vi "UHR-Fleezers Control (host) - 12.0_test_fpga_connection.vi"() -> ()   [LabVIEW 2014] (continued)
        n1069 = Multiply(x=w1416, y=w1429) -> (x*y=w1424:dbl)
        n1070 = Multiply(x=w1428, y=w1415) -> (x*y=w1422:dbl)
        n1071 = Multiply(x=w1427, y=w1414) -> (x*y=w1423:dbl)
        n1072 = Multiply(x=w1430, y=w1413) -> (x*y=w1433:dbl)
        n1073 = Multiply(x=w1431, y=w1412) -> (x*y=w1434:dbl)
        n1074 = Multiply(x=w1432, y=w1411) -> (x*y=w1435:dbl)
        n1075 = call "set RF board amplitude - interlace.vi"("Board 2 Amplitude Limits"=w1397, "Board 1 Amplitude Limits"=w1398, "error in"=w1425, "FPGA VI Reference In"=w1426, "Board 2 Amplitude 3 (%)"=w1435, "Board 1 Amplitude 3 (%)"=w1423, "Board 2 Amplitude 2 (%)"=w1434, "Board 2 Amplitude 1 (%)"=w1433, "Board 1 Amplitude 2 (%)"=w1422, "Board 1 Amplitude 1 (%)"=w1424) -> ("error out"=w1406:errorcluster, "FPGA VI Reference Out"=w1407:T22)
        n1076 = xnode "Read/Write Control"("FPGA VI Reference In"=w1407, "error in"=w1406, "FB On/Off Set 1"=w1402, "FB On/Off Set 2"=w1399) -> ("error out"=w1405:errorcluster)  [unwired: 1 out]
      }
      event "Load parameters": Value Change {
        n1077 = event-data() -> ()  [unwired: 7 out]
        n1078 = property on="Saved AOD Raster Scan Parameter Sets" class="Arr (strict)"() -> ("Index Values"=w1446:u32[])  [unwired: 2 in, 2 out]
        n1079 = Index Array(array=w1446, index=0) -> (element=w1443:u32)
        n1080 = local write "Load parameters"(FALSE ("Load parameters")) -> ()
        n1081 = Index Array(array="Saved AOD Raster Scan Parameter Sets", index=w1443) -> (element=w1442:T31)
        n1082 = Unbundle By Name(w1442) -> ("Scan Range AOD (nm) 2"=w1441:dbl, "Step Size AOD (nm) 2"=w1440:dbl, "Scan Speed AOD (nm/s) 2"=w1439:dbl, "Number of scans (AOD) 2"=w1438:u16)
        n1083 = flat-sequence {
          tunnel: w1441 -> [w1449]
          tunnel: w1440 -> [w1448]
          tunnel: w1439 -> [w1447]
          tunnel: w1438 -> [w1450]
          frame #0 {
            n1084 = local write "Scan Speed (nm/s)"(w1447) -> ()
            n1085 = local write "Scan Range (nm)"(w1449) -> ()
            n1086 = local write "Step Size (nm)"(w1448) -> ()
          }
          frame #1 {
            n1087 = property on="Number of F/B Scans (AOD)" class="DigNum (strict)"("Val(Sgnl)"=w1450) -> ()  [unwired: 2 in, 2 out]
          }
        }
      }
      event "Trap 1 (ON/OFF)", "Trap 2 (ON/OFF)": Value Change {
        n1088 = event-data() -> ()  [unwired: 7 out]
        n1089 = property on="Trap 2 ON" class="Bool (strict)"("Val(Sgnl)"="Trap 2 (ON/OFF)") -> ()  [unwired: 2 in, 2 out]
        n1090 = property on="Trap 1 ON" class="Bool (strict)"("Val(Sgnl)"="Trap 1 (ON/OFF)") -> ()  [unwired: 2 in, 2 out]
      }
      event "DIO count 1 (ticks)", "DIO count 2 (ticks)", "DIO count 3 (ticks)", "Interlace", "Number Interlace Sets", "Not-Interlacing Set": Value Change {
        n1091 = event-data() -> ()  [unwired: 7 out]
        n1092 = local read "DIO count 3 (ticks)"() -> (w1463:u32)
        n1093 = local read "DIO count 1 (ticks)"() -> (w1465:u32)
        n1094 = local read "DIO count 2 (ticks)"() -> (w1464:u32)
        n1095 = To Unsigned Byte Integer(number="Not-Interlacing Set") -> (unsigned 8bit integer=w1454:u8)
        n1096 = Add(x=w1454, y=u8 1) -> (x+y=w1458:u8)
        n1097 = xnode "Read/Write Control"("FPGA VI Reference In"=w1469, "error in"=w1467, "DIO count 1 (ticks)"=w1465, "DIO count 2 (ticks)"=w1464, "DIO count 3 (ticks)"=w1463, "Interlace ON/OFF"="Interlace", "Number Interlace Cycles"="Number Interlace Sets", "Interlace Off Parameters"=w1458) -> ("error out"=w1468:errorcluster)  [unwired: 1 out]
        n1098 = Build Array(w1465, w1464, w1463) -> (w1456:u32[])
        n1099 = Split 1D Array(array=w1456, index="Number Interlace Sets") -> (first subarray=w1466:u32[])  [unwired: 1 out]
        n1100 = Index Array(array=w1456, index=w1454) -> (element=w1455:u32)
        n1101 = Add Array Elements(numeric array=w1466) -> (sum=w1460:u32)
        n1102 = Select(t=w1460, s="Interlace", f=w1455) -> (s? t:f=→"Total Counts (ticks)":u32)
      }
      event "Reset Feedback": Value Change {
        n1103 = event-data() -> ()  [unwired: 7 out]
        n1104 = Unbundle By Name("Reset Feedback") -> ("Set 1"=w1473:bool, "Set 2"=w1472:bool)
        n1105 = xnode "Read/Write Control"("FPGA VI Reference In"=w1475, "error in"=w1470, "FB Reset Set 1"=w1473, "FB Reset Set 2"=w1472) -> ("error out"=w1471:errorcluster)  [unwired: 1 out]
      }
      event "PID Gains": Value Change {
        n1106 = event-data() -> ()  [unwired: 7 out]
        n1107 = Unbundle By Name("PID Gains") -> ("Set 1"=w1479:T15, "Set 2"=w1478:T15)
        n1108 = xnode "Read/Write Control"("FPGA VI Reference In"=w1480, "error in"=w1476, "FB Gains Set 1"=w1479, "FB Gains Set 2"=w1478) -> ("error out"=w1477:errorcluster)  [unwired: 1 out]
      }
      event "AI2 to Setpoint", "Setpoints (V)": Value Change {
        n1109 = event-data() -> ()  [unwired: 7 out]
        n1110 = xnode "Read/Write Control"("FPGA VI Reference In"=w1486, "error in"=w1482) -> ("FPGA VI Reference Out"=w1485:T22, "error out"=w1484:errorcluster, "AI2 Y Sum Set 1"=w1493:i16, "AI2 Y Sum Set 2"=w1492:i16)
        n1111 = Cluster To Array(cluster="AI2 to Setpoint") -> (array=w1496:bool[])
        n1112 = local read "AI2 (V)"() -> (w1494:cluster{"Set 1":dbl, "Set 2":dbl})
        n1113 = Or Array Elements(Boolean array=w1496) -> (logical OR=w1497:bool)
        n1114 = Bundle By Name(cluster=w1494, "Set 1"=w1493, "Set 2"=w1492) -> (w1491:cluster{"Set 1":dbl, "Set 2":dbl})
        n1115 = Divide(x=w1491, y=3276.7) -> (x/y=w1490:cluster{"Set 1":dbl, "Set 2":dbl})
        "AI2 (V)" <- w1490
        n1116 = case shown="True" w1497 {
          tunnel: [w1500 w1517] -> w1489
          tunnel: "AI2 to Setpoint" -> [_ w1513]
          tunnel: "Setpoints (V)" -> [w1501 w1516]
          tunnel: w1490 -> [_ w1510]
          frame False {
            n1117 = Multiply(x=3276.7, y=w1501) -> (x*y=w1502:cluster{"Set 1":dbl, "Set 2":dbl})
            n1118 = To Word Integer(number=w1502) -> (16bit integer=w1500:cluster{"Set 1":i16, "Set 2":i16})
          }
          frame True {
            n1119 = Unbundle By Name(w1510) -> ("Set 1"=w1509:dbl, "Set 2"=w1508:dbl)
            n1120 = Unbundle By Name(w1516) -> ("Set 1"=w1515:dbl, "Set 2"=w1514:dbl)
            n1121 = Unbundle By Name(w1513) -> ("Set 1"=w1512:bool, "Set 2"=w1511:bool)
            n1122 = Select(t=w1509, s=w1512, f=w1515) -> (s? t:f=w1507:dbl)
            n1123 = Select(t=w1508, s=w1511, f=w1514) -> (s? t:f=w1506:dbl)
            n1124 = Bundle By Name(cluster=w1516, "Set 1"=w1507, "Set 2"=w1506) -> (w1504:cluster{"Set 1":dbl, "Set 2":dbl})
            n1125 = local write "Setpoints (V)"(w1504) -> ()
            n1126 = Multiply(x=3276.7, y=w1504) -> (x*y=w1505:cluster{"Set 1":dbl, "Set 2":dbl})
            n1127 = To Word Integer(number=w1505) -> (16bit integer=w1517:cluster{"Set 1":i16, "Set 2":i16})
          }
        }
        n1128 = Unbundle By Name(w1489) -> ("Set 1"=w1488:i16, "Set 2"=w1487:i16)
        n1129 = xnode "Read/Write Control"("FPGA VI Reference In"=w1485, "error in"=w1484, "FB Setpoint Set 1"=w1488, "FB Setpoint Set 2"=w1487) -> ("error out"=w1483:errorcluster)  [unwired: 1 out]
      }
      event "Invert laser interlacing": Value Change {
        n1130 = event-data() -> ()  [unwired: 7 out]
        n1131 = xnode "Read/Write Control"("FPGA VI Reference In"=w1522, "error in"=w1520, "Invert GI"="Invert laser interlacing", "Invert GI 2"="Invert laser interlacing", "Invert RI"="Invert laser interlacing", "Invert RI 2"="Invert laser interlacing") -> ("error out"=w1521:errorcluster)  [unwired: 1 out]
      }
      event "Green FB Setpoint (mV)", "Green FB Gains", "Green FB On/Off", "Green intensity % (FB OFF)", "Green int current ON count adj", "Red intensity % (FB OFF)", "Red FB Gains", "Red FB On/Off", "Red FB Setpoint (mV)": Value Change {
        n1132 = event-data() -> ()  [unwired: 7 out]
        n1133 = local read "Green FB Setpoint (mV)"() -> (w1538:dbl)
        n1134 = local read "Green intensity % (FB OFF)"() -> (w1541:dbl)
        n1135 = local read "Red intensity % (FB OFF)"() -> (w1531:dbl)
        n1136 = local read "Red FB Setpoint (mV)"() -> (w1527:dbl)
        n1137 = Multiply(x=w1527, y=3.2767) -> (x*y=w1525:dbl)
        n1138 = Multiply(x=w1538, y=3.2767) -> (x*y=w1537:dbl)
        n1139 = Multiply(x=w1541, y=655.35) -> (x*y=w1542:dbl)
        n1140 = Multiply(x=w1531, y=655.35) -> (x*y=w1529:dbl)
        n1141 = To Unsigned Word Integer(number=w1542) -> (unsigned 16bit integer=w1540:u16)
        n1142 = To Unsigned Word Integer(number=w1529) -> (unsigned 16bit integer=w1528:u16)
        n1143 = local read "Green int current ON count adj"() -> (w1545:u16)
        n1144 = local read "Green FB Gains"() -> (w1544:T15)
        n1145 = local read "Laser interlacing mode (all lasers)"() -> (w1534:enum32{"Laser ON", "Laser OFF", "Interlace"})
        n1146 = local read "Green ON/Interlacing"() -> (w1535:bool)
        n1147 = local read "Red FB On/Off"() -> (w1524:bool)
        n1148 = local read "Green FB On/Off"() -> (w1546:bool)
        n1149 = local read "Red FB Gains"() -> (w1523:T15)
        n1150 = Equal?(x=w1534, y=enum32{"Laser ON", "Laser OFF", "Interlace"}."Interlace") -> (x = y?=w1532:bool)
        n1151 = Compound Arithmetic op=AND(w1532, w1546, w1535) -> (w1536:bool)
        n1152 = xnode "Read/Write Control"("FPGA VI Reference In"=w1549, "error in"=w1548, "Green FB Setpoint"=w1537, "Green FB On/Off"=w1536, "Current Out"=w1540, "Green int current ON count adj"=w1545, "Green FB Gains"=w1544, "RI Current Out"=w1528, "Red FB Setpoint"=w1525, "Red FB On/Off"=w1524, "Red FB Gains"=w1523) -> ("error out"=w1547:errorcluster)  [unwired: 1 out]
      }
      event "Laser interlacing mode (all lasers)", "Green ON/Interlacing", "Red Laser ON/Interlacing": Value Change {
        n1153 = event-data() -> ()  [unwired: 7 out]
        n1154 = local write "Green Laser ON/OFF"("Green ON/Interlacing") -> ()
        n1155 = case shown="True" "Green ON/Interlacing" {
          tunnel: "Laser interlacing mode (all lasers)" -> [_ w1573]
          tunnel: [enum32{"Laser ON", "Laser OFF", "Interlace"}."Laser OFF" ("Green laser mode") w1573] -> w1556
          tunnel: [FALSE w1569] -> w1555
          frame False {
          }
          frame True {
            n1156 = local read "Green FB On/Off"() -> (w1570:bool)
            n1157 = Equal?(x=w1573, y=enum32{"Laser ON", "Laser OFF", "Interlace"}."Interlace") -> (x = y?=w1571:bool)
            n1158 = And(x=w1571, y=w1570) -> (x .and. y?=w1569:bool)
          }
        }
        n1159 = case shown="True" "Red Laser ON/Interlacing" {
          tunnel: "Laser interlacing mode (all lasers)" -> [_ w1565]
          tunnel: [FALSE w1562] -> w1550
          tunnel: [enum32{"Laser ON", "Laser OFF", "Interlace"}."Laser OFF" ("Green laser mode") w1565] -> w1551
          frame False {
          }
          frame True {
            n1160 = local read "Red FB On/Off"() -> (w1563:bool)
            n1161 = Equal?(x=w1565, y=enum32{"Laser ON", "Laser OFF", "Interlace"}."Interlace") -> (x = y?=w1564:bool)
            n1162 = And(x=w1564, y=w1563) -> (x .and. y?=w1562:bool)
          }
        }
        n1163 = xnode "Read/Write Control"("FPGA VI Reference In"=w1559, "error in"=w1557, "Operating Mode"=w1556, "Operating Mode 2"=w1556, "Green FB On/Off"=w1555, "Red operating mode"=w1551, "RI operating mode 2"=w1551, "Red FB On/Off"=w1550) -> ("error out"=w1558:errorcluster)  [unwired: 1 out]
      }
      event "Green Laser ON/OFF": Value Change {
        n1164 = event-data() -> ()  [unwired: 7 out]
        n1165 = property on="Green ON/Interlacing" class="Bool (strict)"("Val(Sgnl)"="Green Laser ON/OFF") -> ()  [unwired: 2 in, 2 out]
      }
      event "Test ttrig": Value Change {
        n1166 = event-data() -> ()  [unwired: 7 out]
        n1167 = xnode "Read/Write Control"("FPGA VI Reference In"=w1578, "error in"=w1577, "TTrig?"=TRUE) -> ("error out"=w1576:errorcluster)  [unwired: 1 out]
      }
      event "Neg. TTrig FPGA": Value Change {
        n1168 = event-data() -> ()  [unwired: 7 out]
        n1169 = xnode "Read/Write Control"("FPGA VI Reference In"=w1582, "error in"=w1581, "TTrig Negate Pos"="Neg. TTrig FPGA") -> ()  [unwired: 2 out]
      }
      event "- phase (APD 1 Gate)", "+ phase (APD 1 Gate)": Value Change {
        n1170 = event-data() -> ()  [unwired: 7 out]
        n1171 = local read "Phase Adj. (APD 1 Gate)"() -> (w1583:i16)
        n1172 = Negate(x=w1583) -> (-x=w1591:i16)
        n1173 = Select(t=w1591, s="- phase (APD 1 Gate)", f=w1583) -> (s? t:f=w1590:i16)
        n1174 = Or(x="- phase (APD 1 Gate)", y="+ phase (APD 1 Gate)") -> (x .or. y?=w1586:bool)
        n1175 = xnode "Read/Write Control"("FPGA VI Reference In"=w1593, "error in"=w1592, "Phase count adjustment (APD 1 Gate)"=w1590) -> ("FPGA VI Reference Out"=w1588:T22, "error out"=w1589:errorcluster)
        n1176 = xnode "Read/Write Control"("FPGA VI Reference In"=w1588, "error in"=w1589, "+ phase (APD 1 Gate)"=w1586) -> ("error out"=w1587:errorcluster)  [unwired: 1 out]
      }
      event "+ phase (APD 2 Gate)", "- phase (APD 2 Gate)": Value Change {
        n1177 = event-data() -> ()  [unwired: 7 out]
        n1178 = local read "Phase Adj. (APD 2 Gate)"() -> (w1594:i16)
        n1179 = Negate(x=w1594) -> (-x=w1602:i16)
        n1180 = Select(t=w1602, s="- phase (APD 2 Gate)", f=w1594) -> (s? t:f=w1601:i16)
        n1181 = Or(x="- phase (APD 2 Gate)", y="+ phase (APD 2 Gate)") -> (x .or. y?=w1597:bool)
        n1182 = xnode "Read/Write Control"("FPGA VI Reference In"=w1604, "error in"=w1603, "Phase count adjustment (APD 2 Gate)"=w1601) -> ("FPGA VI Reference Out"=w1599:T22, "error out"=w1600:errorcluster)
        n1183 = xnode "Read/Write Control"("FPGA VI Reference In"=w1599, "error in"=w1600, "+ phase (APD 2 Gate)"=w1597) -> ("error out"=w1598:errorcluster)  [unwired: 1 out]
      }
      event "Phase Adj. (APD Acq)", "+ phase (APD Acq)", "- phase (APD Acq)": Value Change {
        n1184 = event-data() -> ()  [unwired: 7 out]
        n1185 = local read "Phase Adj. (APD Acq)"() -> (w1607:i16)
        n1186 = Negate(x=w1607) -> (-x=w1613:i16)
        n1187 = Select(t=w1613, s="+ phase (APD Acq)", f=w1607) -> (s? t:f=w1612:i16)
        n1188 = Or(x="+ phase (APD Acq)", y="- phase (APD Acq)") -> (x .or. y?=w1608:bool)
        n1189 = xnode "Read/Write Control"("FPGA VI Reference In"=w1615, "error in"=w1614, "Phase Count Adjustment (APD Acq)"=w1612) -> ("FPGA VI Reference Out"=w1610:T22, "error out"=w1611:errorcluster)
        n1190 = xnode "Read/Write Control"("FPGA VI Reference In"=w1610, "error in"=w1611, "+ phase (APD Acq)"=w1608) -> ("error out"=w1609:errorcluster)  [unwired: 1 out]
      }
      event "Phase adj. (GI)", "+ phase (GI)", "- phase (GI)", "+phase (RI)", "- phase (RI)", "Phase adj. (RI)": Value Change {
        n1191 = event-data() -> ()  [unwired: 7 out]
        n1192 = Negate(x="Phase adj. (GI)") -> (-x=w1630:i16)
        n1193 = Select(t=w1630, s="+ phase (GI)", f="Phase adj. (GI)") -> (s? t:f=w1629:i16)
        n1194 = Or(x="+ phase (GI)", y="- phase (GI)") -> (x .or. y?=w1625:bool)
        n1195 = Negate(x="Phase adj. (RI)") -> (-x=w1620:i16)
        n1196 = Select(t=w1620, s="+phase (RI)", f="Phase adj. (RI)") -> (s? t:f=w1617:i16)
        n1197 = Or(x="+phase (RI)", y="- phase (RI)") -> (x .or. y?=w1616:bool)
        n1198 = xnode "Read/Write Control"("FPGA VI Reference In"=w1632, "error in"=w1631, "Phase count adjustment (GI)"=w1629, "Phase count adjustment (RI)"=w1617) -> ("FPGA VI Reference Out"=w1627:T22, "error out"=w1628:errorcluster)
        n1199 = xnode "Read/Write Control"("FPGA VI Reference In"=w1627, "error in"=w1628, "+ phase (GI)"=w1625, "+ phase (RI)"=w1616) -> ("error out"=w1626:errorcluster)  [unwired: 1 out]
      }
      event "+ phase (GI) 2", "- phase (GI) 2": Value Change {
        n1200 = event-data() -> ()  [unwired: 7 out]
        n1201 = Negate(x="Phase adj. (GI) 2") -> (-x=w1641:i16)
        n1202 = Select(t=w1641, s="+ phase (GI) 2", f="Phase adj. (GI) 2") -> (s? t:f=w1640:i16)
        n1203 = Or(x="+ phase (GI) 2", y="- phase (GI) 2") -> (x .or. y?=w1636:bool)
        n1204 = xnode "Read/Write Control"("FPGA VI Reference In"=w1643, "error in"=w1642, "Phase count adjustment (GI) 2"=w1640) -> ("FPGA VI Reference Out"=w1638:T22, "error out"=w1639:errorcluster)
        n1205 = xnode "Read/Write Control"("FPGA VI Reference In"=w1638, "error in"=w1639, "+ phase (GI) 2"=w1636) -> ("error out"=w1637:errorcluster)  [unwired: 1 out]
      }
      event "Phase adj. (Green FB)", "- phase (Green FB)", "+ phase (Green FB)": Value Change {
        n1206 = event-data() -> ()  [unwired: 7 out]
        n1207 = Negate(x="Phase adj. (Green FB)") -> (-x=w1652:i16)
        n1208 = Select(t=w1652, s="+ phase (Green FB)", f="Phase adj. (Green FB)") -> (s? t:f=w1651:i16)
        n1209 = Or(x="+ phase (Green FB)", y="- phase (Green FB)") -> (x .or. y?=w1647:bool)
        n1210 = xnode "Read/Write Control"("FPGA VI Reference In"=w1654, "error in"=w1653, "Phase count adjustment (Green FB)"=w1651) -> ("FPGA VI Reference Out"=w1649:T22, "error out"=w1650:errorcluster)
        n1211 = xnode "Read/Write Control"("FPGA VI Reference In"=w1649, "error in"=w1650, "+ phase (Green FB)"=w1647) -> ("error out"=w1648:errorcluster)  [unwired: 1 out]
      }
      event "Invert APD Gate", "APD Gate ON Count", "APD Gate OFF Count", "APD Gate", "APD Integration Time (s)", "APD 1 AO Mult.", "APD 2 AO Mult.", "Duty frequency (ON 1/N cycles)": Value Change {
        n1212 = event-data() -> ()  [unwired: 7 out]
        n1213 = Add(x="Interlace ON count", y="Interlace OFF count") -> (x+y=w1658:u16)
        n1214 = Add(x="APD Gate ON Count", y="APD Gate OFF Count") -> (x+y=w1671:u16)
        n1215 = Multiply(x="Duty frequency (ON 1/N cycles)", y=w1658) -> (x*y=w1657:u16)
        "Green FB Count" <- w1657
        n1216 = Subtract(x=w1657, y="Interlace ON count") -> (x-y=w1655:u16)
        n1217 = Multiply(x=w1671, y="Duty frequency (ON 1/N cycles)") -> (x*y=w1670:u16)
        n1218 = Subtract(x=w1670, y="APD Gate ON Count") -> (x-y=w1669:u16)
        n1219 = local read "DMA Update Period (s)"() -> (w1672:dbl)
        n1220 = Multiply(x="APD Integration Time (s)", y=40000000.0) -> (x*y=w1677:dbl)
        n1221 = Reciprocal(x="APD Integration Time (s)") -> (1/x=→"APD Acq Rate (Hz)":dbl)
        n1222 = To Unsigned Long Integer(number=w1677) -> (unsigned 32bit integer=w1661:u32)
        "APD Int. Count" <- w1661
        n1223 = xnode "Read/Write Control"("FPGA VI Reference In"=w1681, "error in"=w1680, "Invert APD Gate"="Invert APD Gate", "APD Gate ON Count"="APD Gate ON Count", "APD Gate OFF Count"=w1669, "APD Acq Rate Count"=w1661, "APD Gate Operating Mode"="APD Gate", "APD 1 AO scale factor"="APD 1 AO Mult.", "APD 2 AO scale factor"="APD 2 AO Mult.", "Green interlace ON count"="Interlace ON count", "Green interlace OFF count"=w1655, "Green interlace ON count 2"="Interlace ON count", "Green interlace OFF count 2"=w1655, "Green FB Count"=w1657, "RI ON count"="Interlace ON count", "RI OFF count"=w1655) -> ("error out"=w1679:errorcluster)  [unwired: 1 out]
        n1224 = Divide(x=w1672, y="APD Integration Time (s)") -> (x/y=w1675:dbl)
        n1225 = Multiply(x=2.0, y=w1675) -> (x*y=w1674:dbl)
        n1226 = local write "APD Samples/FIFO Acq."(w1675) -> ()
        n1227 = local write "APD Elements/DMA read"(w1674) -> ()
      }
      event "Number of F/B Scans (AOD)", "Scan Speed (nm/s)", "Scan BD", "Initial D (MHz)", "Step Size (nm)", "Scan Range (nm)", "Wiggle amp 1 (units?)": Value Change {
        w1743 = 123.0  # AOM cal (nm/MHz)
        n1228 = event-data() -> ()  [unwired: 7 out]
        n1229 = local read "BD 1 Frequency 1 (MHz)"() -> (w1726:dbl)
        n1230 = local read "AOM X Cal (nm/MHz)"() -> (w1718:dbl)
        n1231 = local read "BD 2 Frequency 1 (MHz)"() -> (w1732:dbl)
        n1232 = local read "X RF Frequency Limits (MHz)"() -> (w1730:T17)
        n1233 = local read "Y RF Frequency Limits (MHz)"() -> (w1727:T17)
        n1234 = Negate(x="Scan Range (nm)") -> (-x=w1696:dbl)
        n1235 = Divide(x=w1696, y=w1718) -> (x/y=w1700:dbl)
        n1236 = Select(t=w1730, s="Scan BD", f=w1727) -> (s? t:f=w1729:T17)
        n1237 = Select(t=w1726, s="Scan BD", f=w1732) -> (s? t:f=w1731:dbl)
        n1238 = Unbundle By Name(w1729) -> ("Maximum"=w1738:dbl, "Minimum"=w1737:dbl)
        n1239 = Add(x=w1700, y=w1731) -> (x+y=w1735:dbl)
        n1240 = Divide(x=w1696, y="Step Size (nm)") -> (x/y=w1715:dbl)
        n1241 = Divide(x="Step Size (nm)", y=w1718) -> (x/y=w1724:dbl)
        n1242 = Absolute Value(x=w1715) -> (abs(x)=w1699:dbl)
        n1243 = Sign(1:w1696) -> (0:w1697:dbl)
        n1244 = In Range and Coerce(upper limit=w1738, x=w1735, lower limit=w1737) -> (coerced(x)=w1734:dbl, In Range?=w1736:bool)
        n1245 = To Unsigned Quad Integer(1:w1699) -> (0:w1714:u64)
        "Scan steps (AOD)" <- w1714
        n1246 = call "IR AOM freq to word.vi"("Frequency In (MHz)"=w1724) -> ("Frequency Word Out (double)"=w1721:dbl)
        n1247 = Multiply(x=w1697, y=w1721) -> (x*y=w1698:dbl)
        n1248 = Subtract(x=w1735, y=w1734) -> (x-y=w1733:dbl)
        n1249 = To Quad Integer(1:w1698) -> (0:w1720:i64)
        "Incr. int (AOD)" <- w1720
        n1250 = Subtract(x=w1700, y=w1733) -> (x-y=w1719:dbl)
        "Scan Range (MHz)" <- w1719
        n1251 = Select(t=w1700, s=w1736, f=w1719) -> (s? t:f=w1739:dbl)
        n1252 = Multiply(x=w1719, y=w1718) -> (x*y=w1717:dbl)
        n1253 = Decrement(x=w1714) -> (x-1=w1767:u64)
        n1254 = Negate(x=w1717) -> (-x=w1713:dbl)
        n1255 = local write "Scan Range (nm)"(w1713) -> ()
        n1256 = Divide(x=w1739, y=w1767) -> (x/y=w1723:dbl)
        "Scan Increment (MHz)" <- w1723
        n1257 = call "IR AOM freq to word.vi"("Frequency In (MHz)"=w1723) -> ("Frequency Word Out (double)"=w1722:dbl)
        n1258 = Divide(x="Step Size (nm)", y="Scan Speed (nm/s)") -> (x/y=w1710:dbl)
        n1259 = To Quad Integer(1:w1722) -> ()  [unwired: 1 out]
        n1260 = local read "Number Interlace Sets"() -> (w1694:u8)
        n1261 = local read "AI Count (ticks)"() -> (w1695:u32)
        n1262 = local read "Total Counts (ticks)"() -> (w1693:u32)
        n1263 = local read "# Samples/trap"() -> (w1725:u32)
        n1264 = Multiply(x=w1695, y=w1694) -> (x*y=w1692:u32)
        n1265 = Divide(x=w1693, y=w1692) -> (x/y=w1691:dbl)
        n1266 = Select(t=w1726, s="Scan BD", f=w1732) -> (s? t:f=w1764:dbl)
        "Initial freq. (MHz)" <- w1764
        n1267 = Add(x=w1739, y=w1764) -> (x+y=→"Final freq. (MHz)":dbl)
        n1268 = Divide(x=w1693, y=40000000.0) -> (x/y=w1709:dbl)
        n1269 = Divide(x=w1710, y=w1709) -> (x/y=w1708:dbl)
        n1270 = To Unsigned Quad Integer(1:w1708) -> (0:w1683:u64)
        n1271 = Quotient & Remainder(x=w1683, y=u64 2) -> (x-y*floor(x/y)=w1687:u64)  [unwired: 1 out]
        n1272 = Equal?(x=w1687, y=u64 0) -> (x = y?=w1685:bool)
        n1273 = Decrement(x=w1683) -> (x-1=w1684:u64)
        n1274 = Select(t=w1683, s=w1685, f=w1684) -> (s? t:f=w1682:u64)
        "Cycles/step (AOD)" <- w1682
        n1275 = xnode "Read/Write Control"("FPGA VI Reference In"=w1775, "error in"=w1774, "Scan steps"=w1714, "Number of scans"="Number of F/B Scans (AOD)", "Cycles per step"=w1682, "Scan freq.  increment"=w1720, "Scan BD"="Scan BD") -> ("error out"=w1773:errorcluster)  [unwired: 1 out]
        n1276 = Multiply(x=w1714, y=w1682) -> (x*y=w1768:u64)
        n1277 = Multiply(x=w1768, y=u64 2) -> (x*y=w1690:u64)
        n1278 = Multiply(x=w1691, y=w1690) -> (x*y=w1689:dbl)
        "Data points/scan (f/b)" <- w1689
        n1279 = Multiply(x=w1689, y="Number of F/B Scans (AOD)") -> (x*y=w1771:dbl)
        "Data points/scans" <- w1771
        n1280 = Divide(x=w1771, y=w1725) -> (x/y=→"N sets should be saved":dbl)
        n1281 = Multiply(x=w1768, y=w1709) -> (x*y=w1707:dbl)
        "Time/Scan (s) (AOD)" <- w1707
        n1282 = Select(t=w1739, s="Scan BD", f=0.0) -> (s? t:f=w1765:dbl)
        n1283 = Select(t=0.0, s="Scan BD", f=w1739) -> (s? t:f=w1761:dbl)
        n1284 = local read "BD 2 Frequency 2 (MHz)"() -> (w1757:dbl)
        n1285 = local read "BD 1 Frequency 2 (MHz)"() -> (w1760:dbl)
        n1286 = Add(x=w1761, y=w1732) -> (x+y=w1758:dbl)
        n1287 = Add(x=w1726, y=w1765) -> (x+y=w1759:dbl)
        n1288 = Multiply(x=w1707, y=2.0) -> (x*y=w1706:dbl)
        n1289 = Multiply(x=w1706, y="Number of F/B Scans (AOD)") -> (x*y=w1703:dbl)
        n1290 = Divide(x=w1703, y=60.0) -> (x/y=→"Time to Finish All (min)":dbl)
        n1291 = Add(x="Trap 2 Bead Size (nm)", y="Trap 1 Bead Size (nm)") -> (x+y=w1747:dbl)
        n1292 = Divide(x=w1747, y=2.0) -> (x/y=w1741:dbl)
        n1293 = Subtract(x=w1758, y=w1757) -> (x-y=w1755:dbl)
        n1294 = Subtract(x=w1759, y=w1760) -> (x-y=w1756:dbl)
        n1295 = local read "Initial D (MHz)"() -> (w1744:dbl)
        n1296 = Square(x=w1755) -> (x^2=w1754:dbl)
        n1297 = Square(x=w1756) -> (x^2=w1753:dbl)
        n1298 = Add(x=w1753, y=w1754) -> (x+y=w1752:dbl)
        n1299 = Square Root(x=w1752) -> (sqrt(x)=w1751:dbl)
        "Final D (MHz)" <- w1751
        n1300 = Multiply(x=w1743, y=w1751) -> (x*y=w1750:dbl)
        n1301 = Multiply(x=w1744, y=w1743) -> (x*y=w1742:dbl)
        n1302 = Subtract(x=w1742, y=w1741) -> (x-y=→"Initial sep (nm)":dbl)
        n1303 = Subtract(x=w1750, y=w1741) -> (x-y=→"Final sep (nm)":dbl)
      }
      event "Freq or Amp switch first", "Swap F1 and F2", "Freq switch delay", "Amp switch delay": Value Change {
        n1304 = event-data() -> ()  [unwired: 7 out]
        n1305 = local read "Freq or Amp switch first"() -> (w1776:bool)
        n1306 = local read "Amp switch delay"() -> (w1777:u16)
        n1307 = local read "Freq switch delay"() -> (w1779:u16)
        n1308 = local read "Swap F1 and F2"() -> (w1778:bool)
        n1309 = xnode "Read/Write Control"("FPGA VI Reference In"=w1782, "error in"=w1781, "Freq switch delay"=w1779, "Swap F1 and F2"=w1778, "Amp switch delay"=w1777, "Freq or Amp switch first"=w1776) -> ("error out"=w1780:errorcluster)  [unwired: 1 out]
      }
      event "Scan steps (MCL)", "Number of scans (MCL)", "Scan Range (V)\n(of steps)", "2D or 1D Scan", "N APD Samp/step", "Fast Scan Dir", "Continuous MCL Scanning", "Scan lines (y)": Value Change {
        w1784 = 32767.0 ("y")
        n1310 = event-data() -> ()  [unwired: 7 out]
        n1311 = Select(t="Scan lines (y)", s="2D or 1D Scan", f="Number of scans (MCL)") -> (s? t:f=w1789:u64)
        n1312 = Decrement(x="Scan steps (MCL)") -> (x-1=w1805:u64)
        n1313 = Divide(x="Scan Range (V)\n(of steps)", y=w1805) -> (x/y=w1804:dbl)
        "Desired Scan Incr (V)" <- w1804
        n1314 = local read "APD Integration Time (s)"() -> (w1797:dbl)
        n1315 = Multiply(x=w1804, y=w1784) -> (x*y=w1813:dbl)
        n1316 = Divide(x=w1813, y=10.0) -> (x/y=w1803:dbl)
        "Desired incr (int)" <- w1803
        n1317 = local read "Update Count (MCL)"() -> (w1809:u32)
        n1318 = Round Toward -Infinity(1:w1803) -> (0:w1812:dbl)
        n1319 = To Word Integer(number=w1812) -> (16bit integer=w1787:i16)
        "Actual Incr. int (MCL)" <- w1787
        n1320 = Multiply(x=w1797, y=40000000.0) -> (x*y=w1810:dbl)
        n1321 = Divide(x=w1810, y=w1809) -> (x/y=w1808:dbl)
        n1322 = Multiply(x=i16 10, y=w1787) -> (x*y=w1785:i16)
        n1323 = Multiply(x="N APD Samp/step", y=w1808) -> (x*y=w1807:dbl)
        "Cycles/step (MCL)" <- w1807
        n1324 = Divide(x=w1785, y=w1784) -> (x/y=→"Actual MCL Inc (V)":dbl)
        n1325 = Multiply(x="N APD Samp/step", y="Scan steps (MCL)") -> (x*y=w1799:dbl)
        n1326 = local read "APD Samples/FIFO Acq."() -> (w1796:dbl)
        n1327 = Multiply(x=w1799, y=u64 2) -> (x*y=w1798:dbl)
        "Data points/scan (f+b)" <- w1798
        n1328 = Multiply(x=w1798, y=w1789) -> (x*y=w1816:dbl)
        "Data points/scans (MCL)" <- w1816
        n1329 = Multiply(x=w1797, y=w1798) -> (x*y=w1790:dbl)
        "Time/f+b scan (s) (MCL)" <- w1790
        n1330 = Divide(x=w1816, y=w1796) -> (x/y=→"N sets should be saved (MCL)":dbl)
        n1331 = Multiply(x=w1790, y=w1789) -> (x*y=→"Total Time (s)":dbl)
        n1332 = Not(x="Fast Scan Dir") -> (.not. x?=w1794:bool)
        n1333 = xnode "Read/Write Control"("FPGA VI Reference In"=w1820, "error in"=w1819, "Scan steps (MCL)"="Scan steps (MCL)", "Number of scans (MCL)"=w1789, "Cycles per step (MCL)"=w1807, "Scan freq.  increment (MCL)"=w1787, "1D or 2D Scan?"="2D or 1D Scan", "MCL Scan Axis"=w1794, "Cont. Scan (MCL)"="Continuous MCL Scanning") -> ("error out"=w1818:errorcluster)  [unwired: 1 out]
      }
      event "Read Cal": Value Change {
        w1822 = 1000.0 ("y")
        n1334 = event-data() -> ()  [unwired: 7 out]
        n1335 = local read "Save file name"() -> (w1847:path)
        n1336 = local write "Read Cal"(FALSE ("Read Cal")) -> ()
        n1337 = Strip Path(path=w1847) -> (stripped path=w1846:path)  [unwired: 1 out]
        n1338 = Path To String(path=w1846) -> (string=w1845:string)
        n1339 = Concatenate Strings(w1845, "\\current.cal" ("string")) -> (w1843:string)
        n1340 = String To Path(string=w1843) -> (path=w1842:path)
        n1341 = Open/Create/Replace File(file path (use dialog)=w1842, operation (0:open)=T30."open", access (0:read/write)=enum16{"read/write", "read-only", "write-only"}."read-only") -> (refnum out=w1850:refnum<file>, error out=w1836:errorcluster)  [unwired: 1 in, 3 out]
        n1342 = Deny Access(4:w1836, 7:w1850) -> (0:w1835:errorcluster, 3:w1841:refnum<file>)  [unwired: 1 out]
        n1343 = Read from Binary File(5:0.0, 8:w1835, 9:T29."big-endian, network order" ("byte order (0:big-endian, network order)"), 10:-1 ("count (1)"), 11:w1841) -> (0:w1834:errorcluster, 2:w1832:dbl[], 3:w1837:refnum<file>)  [unwired: 2 out]
        n1344 = Array To Cluster(array=w1832) -> (cluster=w1831:T32)
        n1345 = Unbundle(w1831) -> ("[0]"=w1830:dbl, "[1]"=w1829:dbl, "[2]"=w1828:dbl, "[3]"=w1827:dbl, "[4]"=w1826:dbl, "[5]"=w1825:dbl)
        n1346 = Close File(refnum=w1837, error in=w1834) -> (error out=→"Read cal error":errorcluster)  [unwired: 1 out]
        n1347 = Multiply(x=w1825, y=w1822) -> (x*y=w1823:dbl)
        n1348 = local write "T2 k_x (pN/nm)"(w1827) -> ()
        n1349 = local write "T1 k_x (pN/nm)"(w1828) -> ()
        n1350 = local write "T1 a_x (nm/V)"(w1830) -> ()
        n1351 = local write "T2 a_x (nm/V)"(w1829) -> ()
        n1352 = Multiply(x=w1826, y=w1822) -> (x*y=w1824:dbl)
        n1353 = local write "T1 offset_x (mV)"(w1824) -> ()
        n1354 = local write "T2 offset_x (mV)"(w1823) -> ()
      }
      event "Read FX file": Value Change {
        n1355 = event-data() -> ()  [unwired: 7 out]
        n1356 = local write "Read FX file"(FALSE ("Read residual")) -> ()
        n1357 = local read "Save file name"() -> (w1875:path)
        n1358 = Strip Path(path=w1875) -> (stripped path=w1874:path)  [unwired: 1 out]
        n1359 = Path To String(path=w1874) -> (string=w1873:string)
        n1360 = Concatenate Strings(w1873, "\\current.cal" ("string")) -> (w1871:string)
        n1361 = String To Path(string=w1871) -> (path=w1870:path)
        n1362 = Open/Create/Replace File(file path (use dialog)=w1870, operation (0:open)=T30."open", access (0:read/write)=enum16{"read/write", "read-only", "write-only"}."read-only") -> (refnum out=w1867:refnum<file>, error out=w1864:errorcluster)  [unwired: 3 in, 1 out]
        n1363 = Deny Access(4:w1864, 7:w1867) -> (0:w1863:errorcluster, 3:w1866:refnum<file>)  [unwired: 1 in]
        n1364 = Read from Binary File(5:0.0, 8:w1863, 9:T29."big-endian, network order" ("byte order (0:big-endian, network order)"), 10:-1 ("count"), 11:w1866) -> (0:w1859:errorcluster, 2:w1853:dbl[], 3:w1860:refnum<file>)  [unwired: 1 in, 1 out]
        n1365 = Index Array(array=w1853, index=6) -> (element=→"Bad fit error":dbl)
        n1366 = Index Array(array=w1853, index=7) -> (element=→"Fit offset":dbl)
        n1367 = Index Array(array=w1853, index=8) -> (element=→"Hyst. error":dbl)
        n1368 = Close File(refnum=w1860, error in=w1859) -> ()  [unwired: 2 out]
      }
      event "Abort MCL Scan": Value Change {
        n1369 = event-data() -> ()  [unwired: 7 out]
        n1370 = local write "MCL Scanning"(FALSE ("MCL Scanning")) -> ()
        n1371 = xnode "Read/Write Control"("FPGA VI Reference In"=w1880, "error in"=w1879, "Abort scan (MCL)"="Abort MCL Scan") -> ("error out"=w1878:errorcluster)  [unwired: 1 out]
      }
      event "Update Count (MCL)": Value Change {
        n1372 = event-data() -> ()  [unwired: 7 out]
        n1373 = xnode "Read/Write Control"("FPGA VI Reference In"=w1884, "error in"=w1883, "MCL count"="Update Count (MCL)") -> ("error out"=w1882:errorcluster)  [unwired: 1 out]
      }
      event "Phase adjust (MCL)", "+ phase (MCL)", "- phase (MCL)": Value Change {
        n1374 = event-data() -> ()  [unwired: 7 out]
        n1375 = Negate(x="Phase adjust (MCL)") -> (-x=w1893:i16)
        n1376 = Select(t=w1893, s="- phase (MCL)", f="Phase adjust (MCL)") -> (s? t:f=w1891:i16)
        n1377 = Or(x="- phase (MCL)", y="+ phase (MCL)") -> (x .or. y?=w1886:bool)
        n1378 = xnode "Read/Write Control"("FPGA VI Reference In"=w1895, "error in"=w1894, "Phase count adjustment (MCL)"=w1891) -> ("FPGA VI Reference Out"=w1887:T22, "error out"=w1888:errorcluster)
        n1379 = xnode "Read/Write Control"("FPGA VI Reference In"=w1887, "error in"=w1888, "+ phase (MCL)"=w1886) -> ("error out"=w1885:errorcluster)  [unwired: 1 out]
      }
      event "Abort AOD Scan": Value Change {
        n1380 = event-data() -> ()  [unwired: 7 out]
        n1381 = xnode "Read/Write Control"("FPGA VI Reference In"=w1899, "error in"=w1898, "Abort scan"="Abort AOD Scan") -> ("error out"=w1897:errorcluster)  [unwired: 1 out]
      }
      event "Continuous AOD Scanning": Value Change {
        n1382 = event-data() -> ()  [unwired: 7 out]
        n1383 = xnode "Read/Write Control"("FPGA VI Reference In"=w1903, "error in"=w1902, "Cont. Scan"="Continuous AOD Scanning") -> ("error out"=w1901:errorcluster)  [unwired: 1 out]
      }
      event "Index": Value Change {
        n1384 = event-data() -> ()  [unwired: 7 out]
        n1385 = call "Create new save file.vi"("Insert"="", "Ext"=".dat" ("string"), "Index In"="Index") -> ("Path Out"=→"Save file name":path, "Index Out"=w1904:dbl)
        "Save index" <- w1904
        n1386 = local write "Index"(w1904) -> ()
      }
      event "AO1", "AO2": Value Change {
        w1919 = 10.0 ("y")
        w1918 = 32767.0 ("y")
        n1387 = event-data() -> ()  [unwired: 7 out]
        n1388 = local read "AO2"() -> (w1917:dbl)
        n1389 = local read "AO1"() -> (w1914:dbl)
        n1390 = Multiply(x=w1914, y=w1918) -> (x*y=w1913:dbl)
        n1391 = Multiply(x=w1917, y=w1918) -> (x*y=w1916:dbl)
        n1392 = Divide(x=w1913, y=w1919) -> (x/y=w1912:dbl)
        n1393 = Divide(x=w1916, y=w1919) -> (x/y=w1915:dbl)
        n1394 = To Word Integer(number=w1912) -> (16bit integer=w1920:i16)
        n1395 = To Word Integer(number=w1915) -> (16bit integer=w1921:i16)
        n1396 = xnode "Read/Write Control"("FPGA VI Reference In"=w1911, "error in"=w1910, "AO1"=w1920, "AO2"=w1921) -> ("error out"=w1909:errorcluster)  [unwired: 1 out]
      }
      event "Inject Pump 1": Value Change {
        n1397 = event-data() -> ()  [unwired: 7 out]
        n1398 = local read "Use Harvard pumps\nfor beads (else Chemyx)"() -> (w1923:bool)
        n1399 = case shown="True" w1923 {
          tunnel: "Inject Pump 1" -> [w1927 w1965]
          tunnel: w1922 -> [_ w1966]
          frame False {
            n1400 = local read "Pump write delay (ms)"() -> (w1926:dbl)
            n1401 = local read "Chemyx Syringe Pump Serial Port"() -> (w1925:refnum<visa-resource-name>)
            n1402 = case shown="True" w1927 {
              tunnel: w1926 -> [w1933 w1947]
              tunnel: w1925 -> [w1930 w1946]
              frame False {
                n1403 = flat-sequence {
                  tunnel: w1930 -> [w1934]
                  tunnel: [w1934] -> w1931
                  tunnel: w1933 -> [_]
                  tunnel: [w1937] -> w1932
                  tunnel: w1931 -> [w1937]
                  tunnel: w1932 -> [w1938]
                  tunnel: [w1938] -> w1928
                  tunnel: [w1940] -> w1929
                  tunnel: w1928 -> [w1940]
                  tunnel: w1929 -> [w1942]
                  frame #0 {
                    n1404 = call "Write to pump.vi"("string"="enter pump1", "VISA resource name"=w1934) -> ()  [unwired: 1 out]
                  }
                  frame #1 {
                    n1405 = Wait (ms)(milliseconds to wait="Pump pause delay (ms)") -> ()  [unwired: 1 out]
                  }
                  frame #2 {
                    n1406 = call "Write to pump.vi"("string"="stop", "VISA resource name"=w1938) -> ()  [unwired: 1 out]
                  }
                  frame #3 {
                    n1407 = Wait (ms)(milliseconds to wait=u32 500) -> ()  [unwired: 1 out]
                  }
                  frame #4 {
                    n1408 = call "Write to pump.vi"("string"="stop", "VISA resource name"=w1942) -> ()  [unwired: 1 out]
                  }
                }
              }
              frame True {
                n1409 = flat-sequence {
                  tunnel: w1946 -> [w1956]
                  tunnel: w1947 -> [w1951]
                  tunnel: w1947 -> [w1958]
                  tunnel: w1946 -> [w1959]
                  tunnel: [w1959] -> w1944
                  tunnel: [w1961] -> w1945
                  tunnel: w1944 -> [w1961]
                  tunnel: w1945 -> [w1963]
                  frame #0 {
                    n1410 = local read "All Pump Parameters"() -> (w1950:T5)
                    n1411 = Unbundle By Name(w1950) -> ("Pump 1"=w1957:T33)
                    n1412 = call "Set pump parameters.vi"("Pump write delay (ms)"=w1951, "Volume (uL)"="Ch 1 Inject Volume (uL)", "Rate (uL/h)"="Ch 1 Inject Rate (ul/h)", "Units"=4.0, "Pump #"=1.0, "Pump Parameters In"=w1957, "VISA resource name"=w1956) -> ("Pump Parameters Out"=w1949:T33)  [unwired: 3 in]
                    n1413 = Bundle By Name(cluster=w1950, "Pump 1"=w1949) -> (w1948:T5)
                    n1414 = local write "All Pump Parameters"(w1948) -> ()
                  }
                  frame #1 {
                    n1415 = Wait (ms)(milliseconds to wait=w1958) -> ()  [unwired: 1 out]
                  }
                  frame #2 {
                    n1416 = call "Write to pump.vi"("string"="start", "VISA resource name"=w1959) -> ()  [unwired: 1 out]
                  }
                  frame #3 {
                    n1417 = Wait (ms)(milliseconds to wait=u32 500) -> ()  [unwired: 1 out]
                  }
                  frame #4 {
                    n1418 = call "Write to pump.vi"("string"="start", "VISA resource name"=w1963) -> ()  [unwired: 1 out]
                  }
                }
              }
            }
          }
          frame True {
            n1419 = case shown="True" w1965 {
              tunnel: w1966 -> [w1967 w1977]
              frame False {
                n1420 = flat-sequence {
                  tunnel: w1967 -> [w1969]
                  frame #0 {
                    n1421 = local write "Flushing P1"(FALSE ("Flushing P1")) -> ()
                    n1422 = Concatenate Strings("stop" ("string"), "\r") -> (w1971:string)
                    n1423 = VISA Write(VISA resource name=w1969, write buffer=w1971) -> ()  [unwired: 1 in, 3 out]
                  }
                  frame #1 {
                    n1424 = property on="Clear Volume P1" class="Bool (strict)"("Val(Sgnl)"=TRUE ("Value (Signaling)")) -> ()  [unwired: 2 in, 2 out]
                  }
                }
              }
              frame True {
                n1425 = local read "Normal Flow Rate (ul/h) P1"() -> (w1975:dbl)
                n1426 = Number To Decimal String(number=w1975) -> (decimal integer string=w1981:string)  [unwired: 1 in]
                n1427 = Concatenate Strings("irate  " ("string"), w1981, " u/h" ("string"), "\r") -> (w1979:string)
                n1428 = VISA Write(VISA resource name=w1977, write buffer=w1979) -> (VISA resource name out=w1976:refnum<visa-resource-name>)  [unwired: 1 in, 2 out]
                n1429 = Concatenate Strings("irun" ("string"), "\r") -> (w1983:string)
                n1430 = VISA Write(VISA resource name=w1976, write buffer=w1983) -> ()  [unwired: 1 in, 3 out]
              }
            }
          }
        }
      }
      event "Inject Pump 3": Value Change {
        n1431 = event-data() -> ()  [unwired: 7 out]
        n1432 = local read "Use Harvard pumps\nfor beads (else Chemyx)"() -> (w1986:bool)
        n1433 = case shown="True" w1986 {
          tunnel: "Inject Pump 3" -> [w1990 w2029]
          tunnel: w1985 -> [_ w2028]
          frame False {
            n1434 = local read "Pump write delay (ms)"() -> (w1989:dbl)
            n1435 = case shown="True" w1990 {
              tunnel: w1989 -> [w1996 w2010]
              tunnel: "Chemyx Syringe Pump Serial Port" -> [w1993 w2009]
              frame False {
                n1436 = flat-sequence {
                  tunnel: w1993 -> [w1997]
                  tunnel: [w1997] -> w1994
                  tunnel: w1996 -> [_]
                  tunnel: [w2000] -> w1995
                  tunnel: w1994 -> [w2000]
                  tunnel: w1995 -> [w2001]
                  tunnel: [w2001] -> w1991
                  tunnel: [w2003] -> w1992
                  tunnel: w1991 -> [w2003]
                  tunnel: w1992 -> [w2005]
                  frame #0 {
                    n1437 = call "Write to pump.vi"("string"="enter pump3", "VISA resource name"=w1997) -> ()  [unwired: 1 out]
                  }
                  frame #1 {
                    n1438 = local read "Pump pause delay (ms)"() -> (w1999:u32)
                    n1439 = Wait (ms)(milliseconds to wait=w1999) -> ()  [unwired: 1 out]
                  }
                  frame #2 {
                    n1440 = call "Write to pump.vi"("string"="stop", "VISA resource name"=w2001) -> ()  [unwired: 1 out]
                  }
                  frame #3 {
                    n1441 = Wait (ms)(milliseconds to wait=u32 0) -> ()  [unwired: 1 out]
                  }
                  frame #4 {
                    n1442 = call "Write to pump.vi"("string"="stop", "VISA resource name"=w2005) -> ()  [unwired: 1 out]
                  }
                }
              }
              frame True {
                n1443 = flat-sequence {
                  tunnel: w2009 -> [w2019]
                  tunnel: w2010 -> [w2014]
                  tunnel: w2010 -> [w2021]
                  tunnel: w2009 -> [w2022]
                  tunnel: [w2022] -> w2008
                  tunnel: [w2025] -> w2007
                  tunnel: w2008 -> [w2025]
                  tunnel: w2007 -> [w2026]
                  frame #0 {
                    n1444 = local read "All Pump Parameters"() -> (w2013:T5)
                    n1445 = Unbundle By Name(w2013) -> ("Pump 3"=w2020:T33)
                    n1446 = call "Set pump parameters.vi"("Pump write delay (ms)"=w2014, "Volume (uL)"="Ch 3 Inject Volume (uL)", "Rate (uL/h)"="Ch 3 Inject Rate (ul/h)", "Units"=4.0, "Pump #"=3.0, "Pump Parameters In"=w2020, "VISA resource name"=w2019) -> ("Pump Parameters Out"=w2012:T33)  [unwired: 3 in]
                    n1447 = Bundle By Name(cluster=w2013, "Pump 3"=w2012) -> (w2011:T5)
                    n1448 = local write "All Pump Parameters"(w2011) -> ()
                  }
                  frame #1 {
                    n1449 = Wait (ms)(milliseconds to wait=w2021) -> ()  [unwired: 1 out]
                  }
                  frame #2 {
                    n1450 = call "Write to pump.vi"("string"="start", "VISA resource name"=w2022) -> ()  [unwired: 1 out]
                  }
                  frame #3 {
                    n1451 = Wait (ms)(milliseconds to wait=u32 500) -> ()  [unwired: 1 out]
                  }
                  frame #4 {
                    n1452 = call "Write to pump.vi"("string"="start", "VISA resource name"=w2026) -> ()  [unwired: 1 out]
                  }
                }
              }
            }
          }
          frame True {
            n1453 = case shown="True" w2029 {
              tunnel: w2028 -> [w2030 w2037]
              frame False {
                n1454 = flat-sequence {
                  tunnel: w2030 -> [w2032]
                  frame #0 {
                    n1455 = local write "Flushing P3"(FALSE ("Flushing P3")) -> ()
                    n1456 = Concatenate Strings("stop" ("string"), "\r") -> (w2034:string)
                    n1457 = VISA Write(VISA resource name=w2032, write buffer=w2034) -> ()  [unwired: 1 in, 3 out]
                  }
                  frame #1 {
                    n1458 = property on="Clear Volume P3" class="Bool (strict)"("Val(Sgnl)"=TRUE ("Value (Signaling)")) -> ()  [unwired: 2 in, 2 out]
                  }
                }
              }
              frame True {
                n1459 = local read "Normal Flow Rate (ul/h) P3"() -> (w2038:dbl)
                n1460 = Number To Decimal String(number=w2038) -> (decimal integer string=w2044:string)  [unwired: 1 in]
                n1461 = Concatenate Strings("irate  " ("string"), w2044, " u/h" ("string"), "\r") -> (w2042:string)
                n1462 = VISA Write(VISA resource name=w2037, write buffer=w2042) -> (VISA resource name out=w2040:refnum<visa-resource-name>)  [unwired: 1 in, 2 out]
                n1463 = Concatenate Strings("irun" ("string"), "\r") -> (w2046:string)
                n1464 = VISA Write(VISA resource name=w2040, write buffer=w2046) -> ()  [unwired: 1 in, 3 out]
              }
            }
          }
        }
      }
      event "Inject Pump 2": Value Change {
        n1465 = event-data() -> ()  [unwired: 7 out]
        n1466 = local read "Pump write delay (ms)"() -> (w2050:dbl)
        n1467 = local read "Chemyx Syringe Pump Serial Port"() -> (w2048:refnum<visa-resource-name>)
        n1468 = flat-sequence {
          tunnel: w2048 -> [w2063]
          tunnel: w2050 -> [w2059]
          tunnel: "Inject Pump 2" -> [_]
          tunnel: w2050 -> [w2065]
          tunnel: w2048 -> [w2066]
          frame #0 {
            n1469 = local read "All Pump Parameters"() -> (w2058:T5)
            n1470 = Multiply(x=60.0, y="Flush Center Ch Rate (ul/m)") -> (x*y=w2055:dbl)
            n1471 = Unbundle By Name(w2058) -> ("Pump 2"=w2064:T33)
            n1472 = call "Set pump parameters.vi"("Pump write delay (ms)"=w2059, "Volume (uL)"="Flush Center Ch Volume (uL)", "Rate (uL/h)"=w2055, "Units"=3.0, "Pump #"=2.0, "Pump Parameters In"=w2064, "VISA resource name"=w2063) -> ("Pump Parameters Out"=w2057:T33)  [unwired: 3 in]
            n1473 = Bundle By Name(cluster=w2058, "Pump 2"=w2057) -> (w2056:T5)
            n1474 = Add(x="Flush Center Ch Volume (uL)", y="Total Volume\nFlushed (uL)") -> (x+y=w2052:dbl)
            n1475 = local write "All Pump Parameters"(w2056) -> ()
            n1476 = local write "Total Volume\nFlushed (uL)"(w2052) -> ()
          }
          frame #1 {
            n1477 = Wait (ms)(milliseconds to wait=w2065) -> ()  [unwired: 1 out]
          }
          frame #2 {
            n1478 = call "Write to pump.vi"("string"="start", "VISA resource name"=w2066) -> ()  [unwired: 1 out]
          }
        }
      }
      event "Sample Channel\nFlow": Value Change {
        n1479 = event-data() -> ()  [unwired: 7 out]
        n1480 = case shown="True" "Sample Channel\nFlow" {
          tunnel: w2069 -> [w2070 w2076]
          frame False {
            n1481 = flat-sequence {
              tunnel: w2070 -> [w2072]
              frame #0 {
                n1482 = local write "Flushing samp"(FALSE ("Flushing samp")) -> ()
                n1483 = Concatenate Strings("stop" ("string"), "\r") -> (w2075:string)
                n1484 = VISA Write(VISA resource name=w2072, write buffer=w2075) -> ()  [unwired: 1 in, 3 out]
              }
            }
          }
          frame True {
            n1485 = local read "Normal Flow rate (mL/h)"() -> (w2086:dbl)
            n1486 = Number To Decimal String(number=w2086) -> (decimal integer string=w2085:string)  [unwired: 1 in]
            n1487 = Concatenate Strings("irate " ("string"), w2085, " u/h" ("string"), "\r") -> (w2081:string)
            n1488 = VISA Write(VISA resource name=w2076, write buffer=w2081) -> (VISA resource name out=w2080:refnum<visa-resource-name>)  [unwired: 1 in, 2 out]
            n1489 = Concatenate Strings("irun" ("string"), "\r") -> (w2077:string)
            n1490 = VISA Write(VISA resource name=w2080, write buffer=w2077) -> ()  [unwired: 1 in, 3 out]
          }
        }
      }
      event "Start Flow": Value Change {
        n1491 = event-data() -> ()  [unwired: 7 out]
        n1492 = local write "Sample Channel\nFlow"(TRUE ("Sample Channel\nFlow")) -> ()
        n1493 = local write "Start Flow"(FALSE ("Start Flow")) -> ()
        n1494 = Concatenate Strings("irun" ("string"), "\r") -> (w2091:string)
        n1495 = VISA Write(VISA resource name=w2087, write buffer=w2091) -> ()  [unwired: 1 in, 3 out]
      }
      event "Stop Flow": Value Change {
        w2093 = FALSE ("Stop Flow")
        n1496 = event-data() -> ()  [unwired: 7 out]
        n1497 = local write "Stop Flow"(w2093) -> ()
        n1498 = local write "Sample Channel\nFlow"(w2093) -> ()
        n1499 = Concatenate Strings("stop" ("string"), "\r") -> (w2096:string)
        n1500 = VISA Write(VISA resource name=w2094, write buffer=w2096) -> ()  [unwired: 1 in, 3 out]
      }
      event "Normal Flow rate (mL/h)": Value Change {
        n1501 = event-data() -> ()  [unwired: 7 out]
        n1502 = Number To Decimal String(number="Normal Flow rate (mL/h)") -> (decimal integer string=w2103:string)  [unwired: 1 in]
        n1503 = Concatenate Strings("irate  " ("string"), w2103, " u/h" ("string"), "\r") -> (w2102:string)
        n1504 = VISA Write(VISA resource name=w2099, write buffer=w2102) -> ()  [unwired: 1 in, 3 out]
      }
      event "Flush Sample": Value Change {
        n1505 = event-data() -> ()  [unwired: 7 out]
        n1506 = flat-sequence {
          tunnel: w2105 -> [w2133]
          frame #0 {
            # "set parameters (rate, volume) for flush, clear volume"
            n1507 = Number To Decimal String(number="Flush rate (mL/m)") -> (decimal integer string=w2129:string)  [unwired: 1 in]
            n1508 = local write "Sample Channel\nFlow"(TRUE ("Sample Channel\nFlow")) -> ()
            n1509 = Concatenate Strings("irate  " ("string"), w2129, " u/m" ("string"), "\r") -> (w2131:string)
            n1510 = VISA Write(VISA resource name=w2133, write buffer=w2131) -> (VISA resource name out=w2127:refnum<visa-resource-name>)  [unwired: 1 in, 2 out]
            n1511 = Number To Decimal String(number="Flush volume (mL)") -> (decimal integer string=w2118:string)  [unwired: 1 in]
            n1512 = Reciprocal(x="Flush rate (mL/m)") -> (1/x=w2112:dbl)
            n1513 = Concatenate Strings("tvolume  " ("string"), w2118, " u" ("string"), "\r") -> (w2116:string)
            n1514 = Multiply(x=w2112, y="Flush volume (mL)") -> (x*y=w2110:dbl)
            n1515 = VISA Write(VISA resource name=w2127, write buffer=w2116) -> (VISA resource name out=w2115:refnum<visa-resource-name>)  [unwired: 1 in, 2 out]
            n1516 = Multiply(x=w2110, y=60.0) -> (x*y=→"Samp Flush Time (s)":dbl)
            n1517 = Concatenate Strings("cvolume" ("string"), "\r") -> (w2114:string)
            n1518 = VISA Write(VISA resource name=w2115, write buffer=w2114) -> (VISA resource name out=w2125:refnum<visa-resource-name>)  [unwired: 1 in, 2 out]
            n1519 = Concatenate Strings("irun" ("string"), "\r") -> (w2123:string)
            n1520 = VISA Write(VISA resource name=w2125, write buffer=w2123) -> ()  [unwired: 1 in, 3 out]
          }
          frame #1 {
            "Flushing samp" <- TRUE ("Boolean")
          }
        }
      }
      event "Flush Pump 3": Value Change {
        n1521 = event-data() -> ()  [unwired: 7 out]
        n1522 = flat-sequence {
          tunnel: w2135 -> [w2138]
          frame #0 {
            # "set paramaters (rate, volume) for flush, clear volume"
            n1523 = Number To Decimal String(number="Flush rate (uL/m) P3") -> (decimal integer string=w2160:string)  [unwired: 1 in]
            n1524 = local write "Inject Pump 3"(TRUE ("Inject Pump 3")) -> ()
            n1525 = Concatenate Strings("irate  " ("string"), w2160, " u/m" ("string"), "\r") -> (w2162:string)
            n1526 = VISA Write(VISA resource name=w2138, write buffer=w2162) -> (VISA resource name out=w2158:refnum<visa-resource-name>)  [unwired: 1 in, 2 out]
            n1527 = Reciprocal(x="Flush rate (uL/m) P3") -> (1/x=w2142:dbl)
            n1528 = Number To Decimal String(number="Volume (uL) P3") -> (decimal integer string=w2149:string)  [unwired: 1 in]
            n1529 = Multiply(x="Volume (uL) P3", y=w2142) -> (x*y=w2141:dbl)
            n1530 = Concatenate Strings("tvolume  " ("string"), w2149, " u" ("string"), "\r") -> (w2147:string)
            n1531 = Multiply(x=w2141, y=60.0) -> (x*y=→"HP3 Flush Time (s)":dbl)
